vi "PWM CAP Stop.vi"(8 "error in (no error)":errorcluster, 10 "Channel":u8, 11 "DevHandle":i32) -> (0 "error out":errorcluster, 3 "function return":i32)   [LabVIEW 2010, in "usb2pwm.lvlib"]
doc: "int WINAPI PWM_CAP_Stop(int DevHandle, unsigned char Channel);"
uses:
  usb2pwm.lvlib
  libs/msvc_x86/USB2XXX.dll
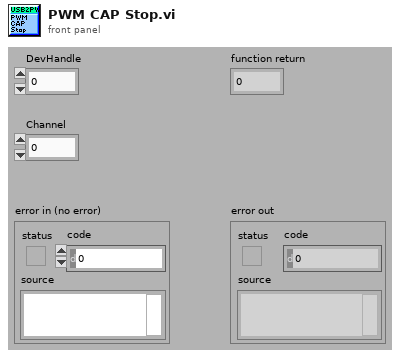
[diagram p1: front panel]
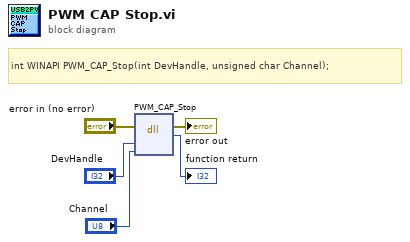
[diagram p0: block diagram]
diagram:
  # "int WINAPI PWM_CAP_Stop(int DevHandle, unsigned char Channel);"
  n1 = dll-call lib="E:/OtherWork/STM32/USB2XXX_Example/sdk/libs/msvc_x86/USB2XXX.*" fn="PWM_CAP_Stop"(error in="error in (no error)", "DevHandle"="DevHandle", "Channel"="Channel") -> (error out=→"error out":errorcluster, →"function return":i32)  [unwired: 4 in, 1 out]
